vi "On Context Menu Requested.vi"(8 "error in (no error)":errorcluster, 10 "Data":T1, 11 "WebView2 Event Filter Interface in":refnum<class "WebView2 Event Filter Interface.lvclass">) -> (0 "error out":errorcluster, 1 "SelectedCommandId":i32, 2 "Handled":bool)   [LabVIEW 2025, in "WebView2.lvlib" / "WebView2 Event Filter Interface.lvclass"]
uses:
  WebView2 Event Filter Interface.lvclass
  WebView2 Control Object/Context Menu Requested Event Data.ctl
  E:/Labview/LV 2023/PPL/PPL Builder/Libs/LV-WebView2/Source/Libs/Microsoft.Web.WebView2.Core.dll
  Libs/Microsoft.Web.WebView2.Core.dll
  System.Drawing
  WebView2 Control Object/WebView2 Control.lvclass
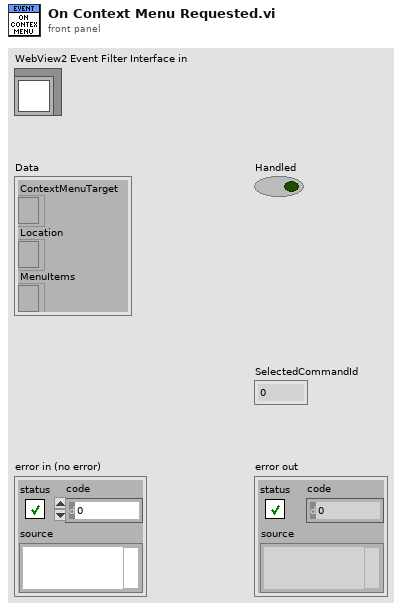
[diagram p1: front panel]
types:
  T1 = typedef "WebView2.lvlib/WebView2 Control.lvclass/Context Menu Requested Event Data.ctl" = cluster{"ContextMenuTarget":refnum<k24>, "Location":refnum<k24>, "MenuItems":refnum<k24>}
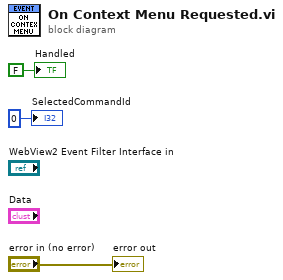
[diagram p0: block diagram]
diagram:
  "error out" <- "error in (no error)"
  "SelectedCommandId" <- 0 ("SelectedCommandId")
  "Handled" <- FALSE ("Handled")
